vi "Create New Handler with Console.vi"(6 "Show Console":bool=TRUE, 7 "Handler.UserEvent.Console in":refnum<class "Handler.UserEvent.Console.lvclass">, 8 "error in (no error)":errorcluster, 10 "Name":string, 11 "Level":T1(ring)) -> (0 "error out":errorcluster, 3 "Handler.UserEvent.Console out":refnum<class "Handler.UserEvent.Console.lvclass">)   [LabVIEW 2017, in "Error Log.lvlib" / "Handler.UserEvent.Console.lvclass"]
uses:
  Handler.UserEvent.Console.lvclass
  \\192.168.1.40\Neosoft/Partage/Dossiers Personnels/BRO/DevTools_BR/wc/ErrorLog/src/Handler/Handler.lvclass
  Handler/Handler.lvclass
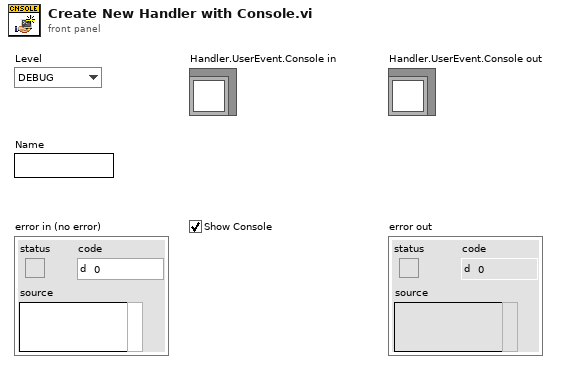
[diagram p1: front panel]
types:
  T1 = enum16{"DEBUG", "INFO", "WARNING", "ERROR", "CRITICAL"}
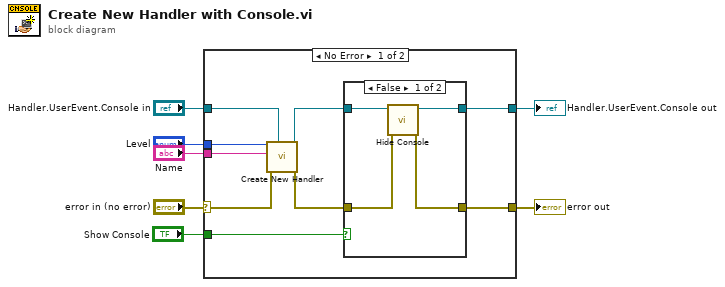
[diagram p0: block diagram]
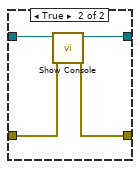
[diagram p2: hidden frame]
diagram:
  n1 = case shown="No Error" "error in (no error)" {
    selector: "error in (no error)" -> [w16 w26]
    tunnel: [w9 w26] -> w6
    tunnel: [w11 w25] -> w4
    tunnel: "Handler.UserEvent.Console in" -> [w15 w25]
    tunnel: "Level" -> [w14 _]
    tunnel: "Name" -> [w13 _]
    tunnel: "Show Console" -> [w8 _]
    frame No Error {
      n2 = call "Create New Handler.vi"("Handler type"=w15, "error in (no error)"=w16, "Name"=w13, "Level"=w14) -> ("error out"=w10:errorcluster, "Handler"=w12:refnum<class "Handler.UserEvent.Console.lvclass">)  [unwired: 6 in]
      n3 = case shown="False" w8 {
        tunnel: w12 -> [w20 w24]
        tunnel: [w19 w23] -> w11
        tunnel: w10 -> [w18 w22]
        tunnel: [w17 w21] -> w9
        frame False {
          n4 = call "Hide Console.vi"("error in (no error)"=w18, "Handler.UserEvent.Console in"=w20) -> ("error out"=w17:errorcluster, "Handler.UserEvent.Console out"=w19:refnum<class "Handler.UserEvent.Console.lvclass">)  [unwired: 8 in]
        }
        frame True {
          n5 = call "Show Console.vi"("error in (no error)"=w22, "Handler.UserEvent.Console in"=w24) -> ("error out"=w21:errorcluster, "Handler.UserEvent.Console out"=w23:refnum<class "Handler.UserEvent.Console.lvclass">)  [unwired: 8 in]
        }
      }
    }
    frame Error {
    }
  }
  "error out" <- w6
  "Handler.UserEvent.Console out" <- w4
